vi "HMI Main.vi"() -> ()   [LabVIEW 2014]
uses:
  Type Def/HMI State Machine.ctl
panel:
  in  "Trend screen":bool
  in  "Settings":bool
  in  "exit":bool
  in  "Tab Control":enum32{"Operations", "Trend", "Settings"}(tab)
  in  "Zero":bool
  in  "Hold":bool
  out "Bit Load [lbs]":dbl
  out "Bit RPM":dbl
  out "BH Limit Point Read":dbl caption="Block Hight Limit" format="%.1f"
  out "Torque Limit Point Read":dbl caption="Torque Limit" format="%.1f"
  out "Torque Bar":dbl(slide) scale=0.0..100.0
  out "RPM Point Read":dbl caption="RPM Setpoint\n[RPM]" format="%.1f"
  out "WOB Point Read":dbl caption="WOB Setpoint" format="%.1f"
  out "ROP Point Read":dbl caption="ROP Setpoint \n[in/min]" format="%.1f"
  in  "stop":bool
  in  "Run":bool
  out "WOB Gauge":dbl(knob) scale=0.0..100.0 scale format="%#_4g"
  out "RPM Gauge":dbl(knob) scale=0.0..100.0 scale format="%#_4g"
  out "ROP Gauge":dbl(knob) scale=0.0..100.0 scale format="%#_4g"
  out "BH Bar":dbl(slide) scale=0.0..100.0
  in  "Log":bool
  out "ROP/WOB Chart":T1(graph)
  out "Torq/RPM Chart":T2(graph)
  in  "Back to Main 9":bool
  in  "Back to Main 3":bool
  out "Time":timestamp format="%<%X>T"
  # "Block Position"
  # "Torque"
  # "WOB"
  # "ROP"
  # "RPM"
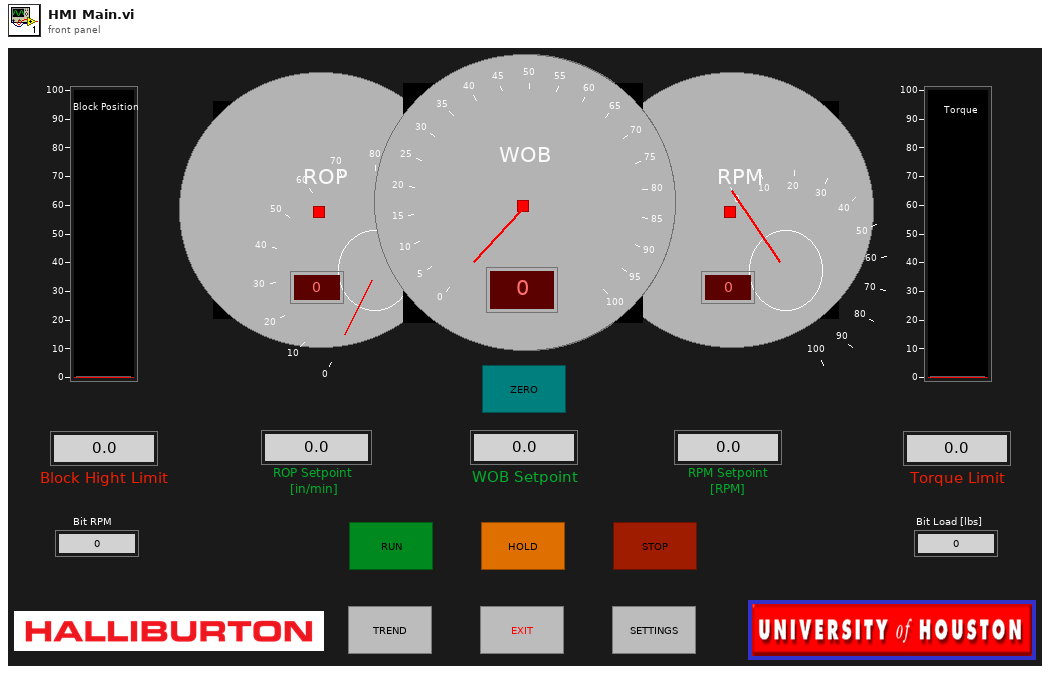
[diagram p1: front panel]
types:
  T1 = cluster{"Bit RPM":dbl, "Bit RPM":dbl, "Bit RPM":dbl, "Bit RPM":dbl, "Double":dbl}
  T2 = cluster{"Bit RPM":dbl, "Bit RPM":dbl, "Bit RPM":dbl, "Double":dbl}
  T3 = typedef "HMI State Machine.ctl" = enum16{"Init", "Run", "Exit"}
  T4 = cluster{"left":i16, "top":i16, "right":i16, "bottom":i16}
  T5 = cluster{"Bit RPM":dbl, "Double":dbl, "Double":dbl, "Double":dbl}
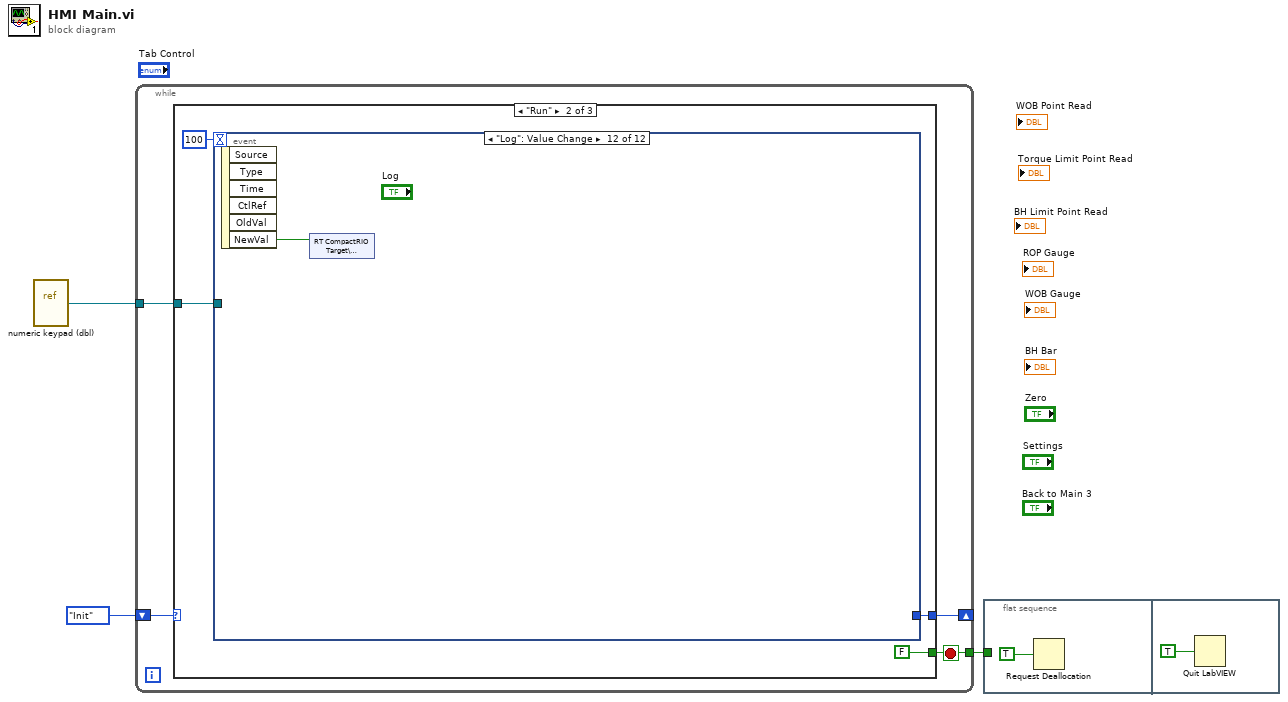
[diagram p0: block diagram]
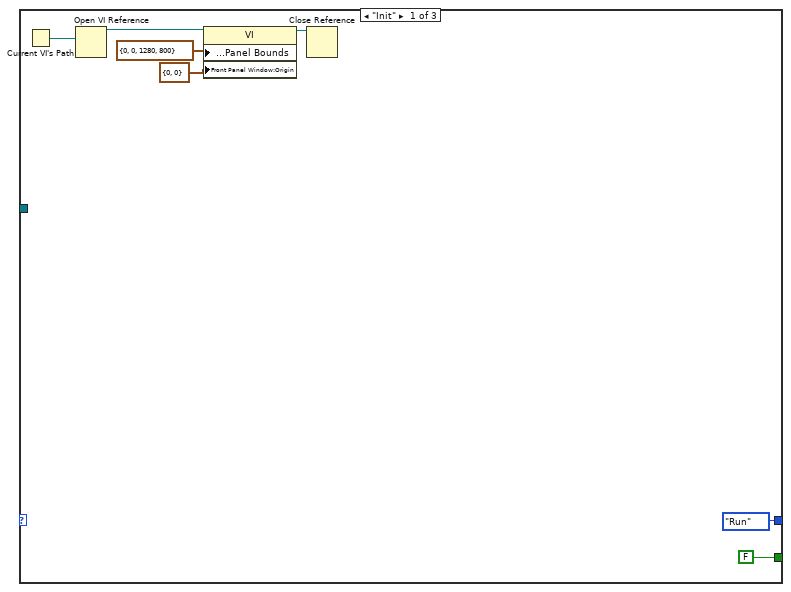
[diagram p2: hidden frame]
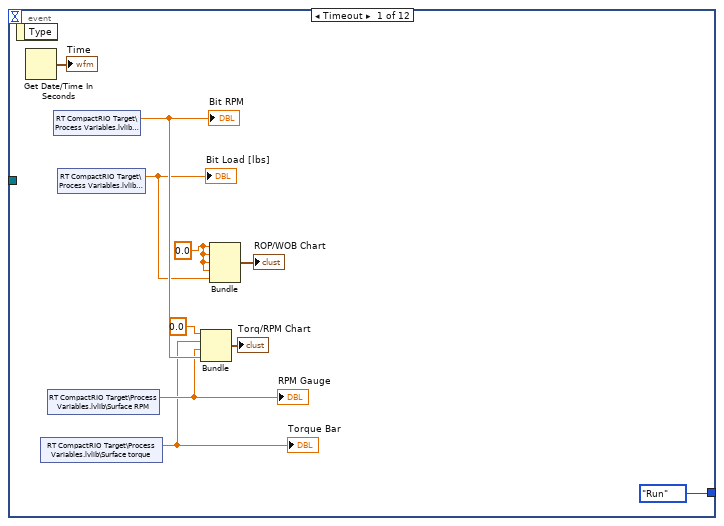
[diagram p3: hidden frame]
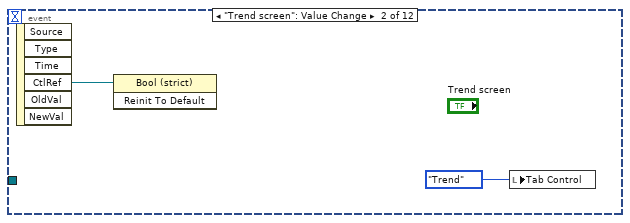
[diagram p4: hidden frame]
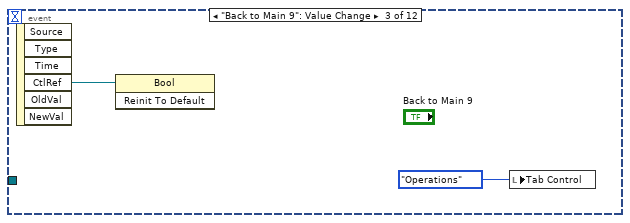
[diagram p5: hidden frame]
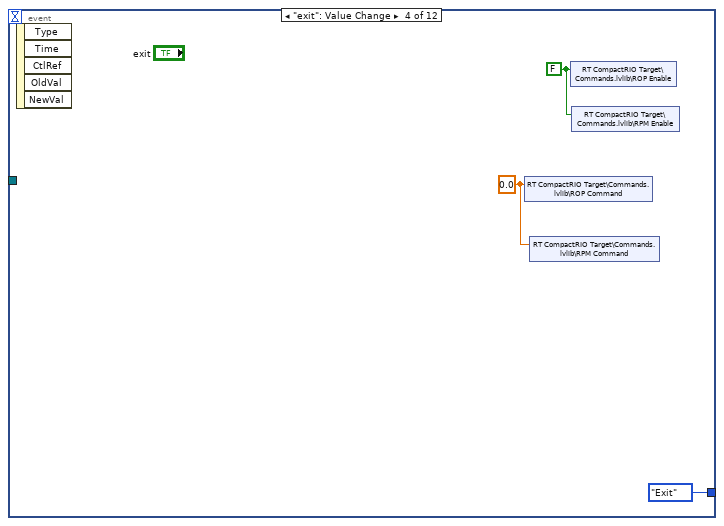
[diagram p6: hidden frame]
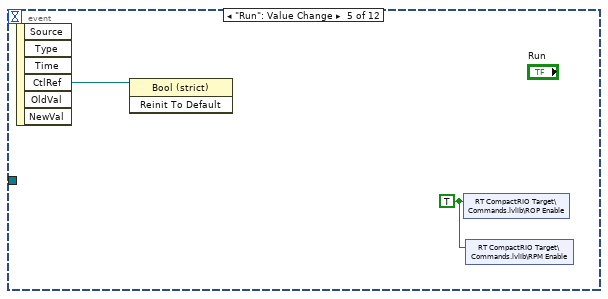
[diagram p7: hidden frame]
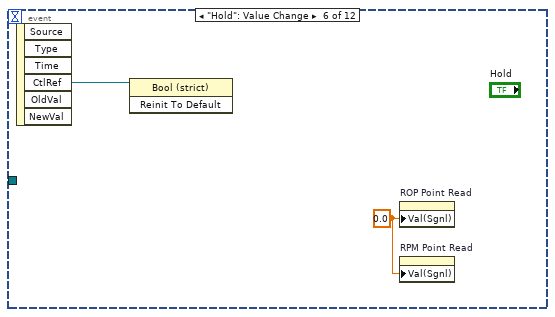
[diagram p8: hidden frame]
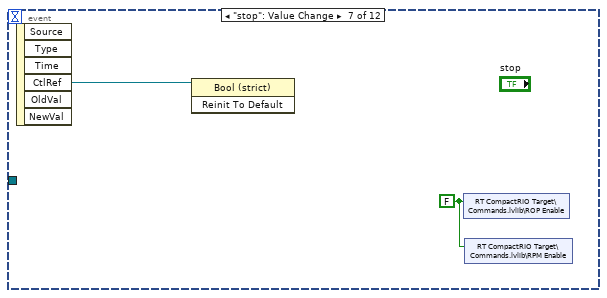
[diagram p9: hidden frame]
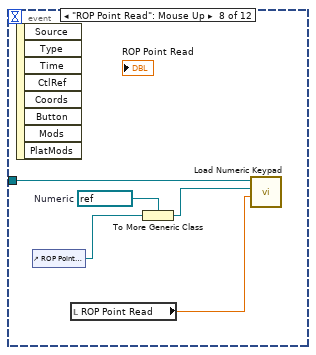
[diagram p10: hidden frame]
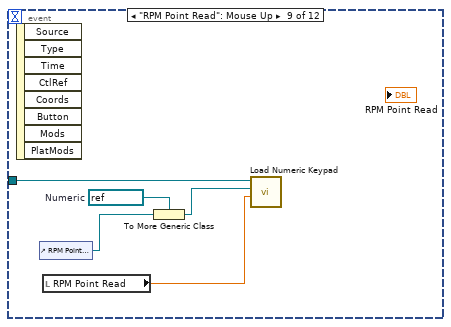
[diagram p11: hidden frame]
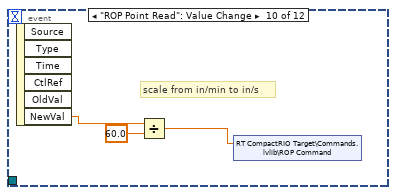
[diagram p12: hidden frame]
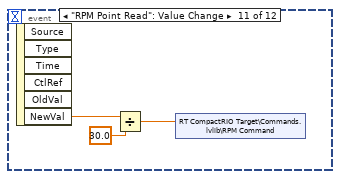
[diagram p13: hidden frame]
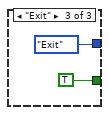
[diagram p14: hidden frame]
diagram:
  n1 = vi-ref "numeric keypad (dbl).vi"() -> (w1:refnum<vi>)
  n2 = while {
    shift-right: [w6] -> _
    shift-left: HMI_State_Machine."Init" ("HMI State Machine") -> [w7]
    tunnel: [w5] -> w2
    tunnel: w1 -> [w4]
    stop <- w5 stop-if-true
    n3 = case shown="\"Run\"" w7 {
      tunnel: [HMI_State_Machine."Run" ("HMI State Machine") w16 HMI_State_Machine."Exit" ("HMI State Machine")] -> w6
      tunnel: [FALSE FALSE TRUE] -> w5
      tunnel: w4 -> [_ w15 _]
      frame "Init" {
        n4 = Current VI's Path() -> (path=w8:path)
        n5 = Open VI Reference(vi path=w8) -> (vi reference=w12:refnum<vi>)  [unwired: 5 in, 1 out]
        n6 = property class="VI"(reference=w12, "Front Panel Window:Panel Bounds"=T4 {"left"=0, "top"=0, "right"=1280, "bottom"=800}, "Front Panel Window:Origin"=cluster{"Horizontal":i16, "Vertical":i16} {"Horizontal"=0, "Vertical"=0}) -> (reference out=w9:refnum<vi>)  [unwired: 1 in, 1 out]
        n7 = Close Reference(reference=w9) -> ()  [unwired: 1 in, 1 out]
      }
      frame "Run" {
        n8 = event shown="[11] \"Log\": Value Change" {
          selector: _ -> [_ _ _ _ _ _ _ _ _ _ _ _]
          dyn-events: _ -> [_ _ _ _ _ _ _ _ _ _ _ _]
          timeout: 100 -> [_ _ _ _ _ _ _ _ _ _ _ _]
          tunnel: [HMI_State_Machine."Run" ("HMI State Machine") _ _ HMI_State_Machine."Exit" ("HMI State Machine") _ _ _ _ _ _ _ _] -> w16
          tunnel: w15 -> [_ _ _ _ _ _ _ w46 w51 _ _ _]
          event Timeout {
            w22 = 0.0 ("Bit RPM")
            n9 = event-data() -> ()  [unwired: 1 in, 1 out]
            n10 = Get Date/Time In Seconds() -> (seconds since 1Jan1904=→"Time":timestamp)
            n11 = shared-variable "RT CompactRIO Target\\Process Variables.lvlib\\Surface torque"() -> (w19:dbl)  [unwired: 1 in, 1 out]
            "Torque Bar" <- w19
            n12 = shared-variable "RT CompactRIO Target\\Process Variables.lvlib\\Surface RPM"() -> (w20:dbl)  [unwired: 1 in, 1 out]
            "RPM Gauge" <- w20
            n13 = shared-variable "RT CompactRIO Target\\Process Variables.lvlib\\Bit RPM"() -> (w26:dbl)  [unwired: 1 in, 1 out]
            "Bit RPM" <- w26
            n14 = shared-variable "RT CompactRIO Target\\Process Variables.lvlib\\Bit Load"() -> (w21:dbl)  [unwired: 1 in, 1 out]
            "Bit Load [lbs]" <- w21
            n15 = Bundle("Bit RPM"=0.0, "Double"=w19, "Double"=w20, "Double"=w26) -> (→"Torq/RPM Chart":T5)  [unwired: 1 in]
            n16 = Bundle("Bit RPM"=w22, "Bit RPM"=w22, "Bit RPM"=w22, "Bit RPM"=w22, "Double"=w21) -> (→"ROP/WOB Chart":T1)  [unwired: 1 in]
          }
          event "Trend screen": Value Change {
            n17 = event-data() -> ("CtlRef"=w29:refnum<vi>)  [unwired: 1 in, 5 out]
            n18 = invoke class="Bool (strict)" method="Reinit To Default"(reference=w29) -> ()  [unwired: 2 in, 3 out]
            n19 = local write "Tab Control"(enum32{"Operations", "Trend", "Settings"}."Trend" ("Tab Control")) -> ()
          }
          event "Back to Main 9": Value Change {
            n20 = event-data() -> ("CtlRef"=w31:refnum<vi>)  [unwired: 1 in, 5 out]
            n21 = invoke class="Bool" method="Reinit To Default"(reference=w31) -> ()  [unwired: 2 in, 3 out]
            n22 = local write "Tab Control"(enum32{"Operations", "Trend", "Settings"}."Operations" ("Tab Control")) -> ()
          }
          event "exit": Value Change {
            w33 = 0.0 ("ROP Command")
            w34 = FALSE ("ROP Enable")
            n23 = event-data() -> ()  [unwired: 1 in, 5 out]
            n24 = shared-variable "RT CompactRIO Target\\Commands.lvlib\\ROP Command"(w33) -> ()  [unwired: 1 in, 1 out]
            n25 = shared-variable "RT CompactRIO Target\\Commands.lvlib\\RPM Command"(w33) -> ()  [unwired: 1 in, 1 out]
            n26 = shared-variable "RT CompactRIO Target\\Commands.lvlib\\ROP Enable"(w34) -> ()  [unwired: 1 in, 1 out]
            n27 = shared-variable "RT CompactRIO Target\\Commands.lvlib\\RPM Enable"(w34) -> ()  [unwired: 1 in, 1 out]
          }
          event "Run": Value Change {
            w37 = TRUE ("ROP Enable")
            n28 = event-data() -> ("CtlRef"=w36:refnum<vi>)  [unwired: 1 in, 5 out]
            n29 = invoke class="Bool (strict)" method="Reinit To Default"(reference=w36) -> ()  [unwired: 2 in, 3 out]
            n30 = shared-variable "RT CompactRIO Target\\Commands.lvlib\\ROP Enable"(w37) -> ()  [unwired: 1 in, 1 out]
            n31 = shared-variable "RT CompactRIO Target\\Commands.lvlib\\RPM Enable"(w37) -> ()  [unwired: 1 in, 1 out]
          }
          event "Hold": Value Change {
            w38 = 0.0 ("Value (Signaling)")
            n32 = event-data() -> ("CtlRef"=w39:refnum<vi>)  [unwired: 1 in, 5 out]
            n33 = invoke class="Bool (strict)" method="Reinit To Default"(reference=w39) -> ()  [unwired: 2 in, 3 out]
            n34 = property on="ROP Point Read" class="DigNum (strict)"("Val(Sgnl)"=w38) -> ()  [unwired: 2 in, 2 out]
            n35 = property on="RPM Point Read" class="DigNum (strict)"("Val(Sgnl)"=w38) -> ()  [unwired: 2 in, 2 out]
          }
          event "stop": Value Change {
            w41 = FALSE ("ROP Enable")
            n36 = event-data() -> ("CtlRef"=w40:refnum<vi>)  [unwired: 1 in, 5 out]
            n37 = invoke class="Bool (strict)" method="Reinit To Default"(reference=w40) -> ()  [unwired: 2 in, 3 out]
            n38 = shared-variable "RT CompactRIO Target\\Commands.lvlib\\ROP Enable"(w41) -> ()  [unwired: 1 in, 1 out]
            n39 = shared-variable "RT CompactRIO Target\\Commands.lvlib\\RPM Enable"(w41) -> ()  [unwired: 1 in, 1 out]
          }
          event "ROP Point Read": Mouse Up {
            w44 = refnum<vi> refnum  # Numeric
            n40 = event-data() -> ()  [unwired: 1 in, 8 out]
            n41 = control-ref of="ROP Point Read"() -> (w42:refnum<vi>)
            n42 = local read "ROP Point Read"() -> (w45:dbl)
            n43 = To More Generic Class(target class=w44, reference=w42) -> (generic class reference=w43:refnum<vi>)
            n44 = call "Load Numeric Keypad.vi"("Initial Value"=w45, "Numeric ctrlRef"=w43, "VI Refnum"=w46) -> ()  [unwired: 8 in, 1 out]
          }
          event "RPM Point Read": Mouse Up {
            w49 = refnum<vi> refnum  # Numeric
            n45 = event-data() -> ()  [unwired: 1 in, 8 out]
            n46 = control-ref of="RPM Point Read"() -> (w47:refnum<vi>)
            n47 = local read "RPM Point Read"() -> (w50:dbl)
            n48 = To More Generic Class(target class=w49, reference=w47) -> (generic class reference=w48:refnum<vi>)
            n49 = call "Load Numeric Keypad.vi"("Initial Value"=w50, "Numeric ctrlRef"=w48, "VI Refnum"=w51) -> ()  [unwired: 8 in, 1 out]
          }
          event "ROP Point Read": Value Change {
            # "scale from in/min to in/s"
            n50 = event-data() -> ("NewVal"=w53:dbl)  [unwired: 1 in, 5 out]
            n51 = Divide(x=w53, y=60.0) -> (x/y=w54:dbl)
            n52 = shared-variable "RT CompactRIO Target\\Commands.lvlib\\ROP Command"(w54) -> ()  [unwired: 1 in, 1 out]
          }
          event "RPM Point Read": Value Change {
            n53 = event-data() -> ("NewVal"=w57:dbl)  [unwired: 1 in, 5 out]
            n54 = Divide(x=w57, y=30.0) -> (x/y=w56:dbl)
            n55 = shared-variable "RT CompactRIO Target\\Commands.lvlib\\RPM Command"(w56) -> ()  [unwired: 1 in, 1 out]
          }
          event "Log": Value Change {
            n56 = event-data() -> ("NewVal"=w58:bool)  [unwired: 1 in, 5 out]
            n57 = shared-variable "RT CompactRIO Target\\Commands.lvlib\\Log"(w58) -> ()  [unwired: 1 in, 1 out]
          }
        }
      }
      frame "Exit" {
      }
    }
  }
  n58 = flat-sequence {
    tunnel: w2 -> [_]
    frame #0 {
      n59 = Request Deallocation(TRUE ("flag")) -> ()
    }
    frame #1 {
      n60 = Quit LabVIEW(quit? (T)=TRUE) -> ()
    }
  }
